vi "Set Build Specification Name.vi"(8 "error in (no error)":errorcluster, 10 "Build Specification Name":string, 11 "NI_AB_API_Build in":refnum<class "NI_AB_API_Build.lvclass">) -> (0 "error out":errorcluster, 3 "NI_AB_API_Build out":refnum<class "NI_AB_API_Build.lvclass">)   [LabVIEW 2020, in "NI_AB_API_Build.lvclass"]
uses:
  <vilib>/AppBuilder/AB_API/Build/NI_AB_API_Build.lvclass
  <vilib>/AppBuilder/AB_API/Build/NI_AB_API_Build.lvclass/NI_AB_API_Build.ctl
  <resource>/Framework/Providers/API/mxLvUpdateUI.ctl
  <vilib>/AppBuilder/AB_Classes/Build/AB_Build.lvclass
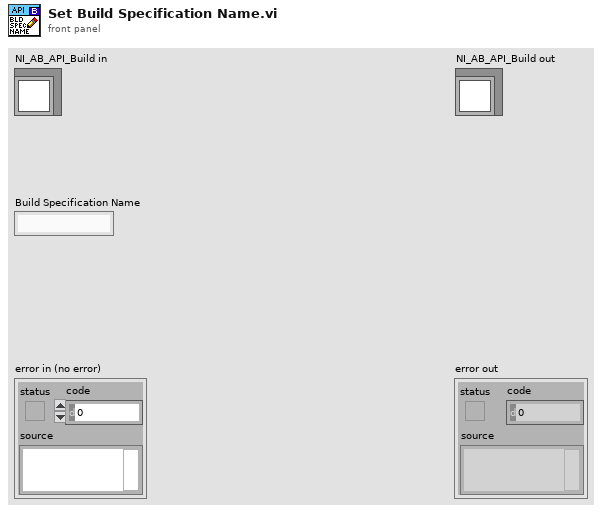
[diagram p1: front panel]
types:
  T1 = typedef "mxLvUpdateUI.ctl" = cluster{"Action":u32, "Optional param 1":string, "Optional param 2":i32, "Optional param 3":string}
  T2 = typedef "AB_Build.ctl" = cluster{"buildSpecName":string, "buildSpecDescription":string, "destinations":refnum<class "AB_Destination.lvclass">[], "exclusionOption":T3, "defaultLanguage":string, "supportedLanguages":string[], "excludedDirectories":path[], "buildContext":refnum<vi>, "buildObject":T4, "preview":bool, "programatic":bool, "progressBarEvents":T5, "userLog_Path":path, "preActionID":string, "preAction_Path":path, "postActionID":string, "postAction_Path":path, "eng_checkForBrokenVIs?":bool, "eng_verboseLinkerErrors?":bool, "localDest_Path":path, "targetDest_Path":path, "removeVIObject":u16, "cache":refnum<class "PreviewCache.lvclass">, "use cache":bool, "previewCache_ID":string, "buildCache_ID":string, "eng_TempLocalDest_Path":path, "eng_collectDependencies?":bool, "versionInfo":cluster{"buildVersion":cluster{"major":u16, "minor":u16, "patch":u16, "build":u16}, "autoIncrement":bool}, "eng_enableVIChecksums":bool}
  T3 = typedef "AB_Exclusion_Option.ctl" = cluster{"typedefs":bool, "polymorphicVIs":bool, "unusedLibraryItems":bool, "modifyLibraryFile":bool, "edit-timeDependencies":bool, "inlineVIs":bool, "dependent PPLs":bool, "dependent DLLs":bool}
  T4 = typedef "ItemRef.ctl" = u64
  T5 = typedef "provcom_ProgressBar_Events.ctl" = cluster{"newJob":refnum<user-event>, "newItem":refnum<user-event>, "errorMsg":T6, "cancel":refnum<user-event>}
  T6 = typedef "mxLvBuildError.ctl" = refnum<user-event>
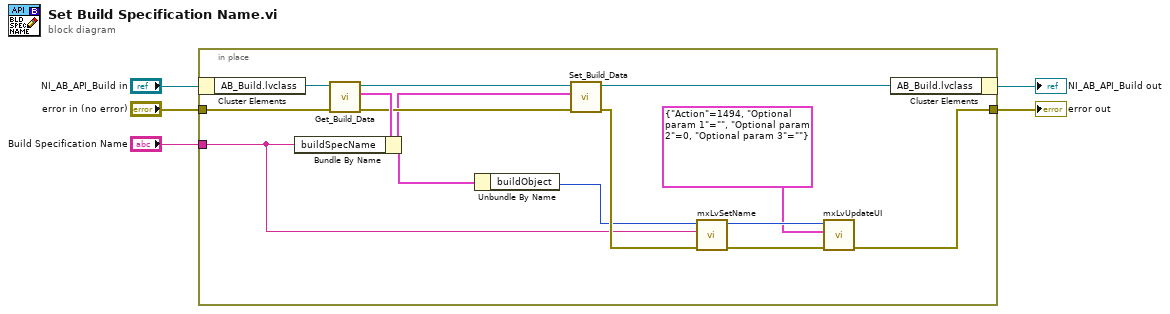
[diagram p0: block diagram]
diagram:
  n1 = in-place {
    in-place-border: [w11] -> w4
    in-place-border: "error in (no error)" -> [w19]
    in-place-border: "Build Specification Name" -> [w6]
    n2 = in-place-cluster #1("NI_AB_API_Build in") -> ("AB_Build.lvclass"=w14:refnum<class "AB_Build.lvclass">)
    n3 = call <vilib>:"Get_Build_Data.vi"("error in (no error)"=w19, "Class in"=w14) -> ("error out"=w16:errorcluster, "data"=w17:T2, "Class out"=w18:refnum<class "AB_Build.lvclass">)  [unwired: 7 out]
    n4 = Bundle By Name(cluster=w17, "buildSpecName"=w6) -> (w13:T2)
    n5 = Unbundle By Name(w13) -> ("buildObject"=w10:T4)
    n6 = call <vilib>:"Set_Build_Data.vi"("error in (no error)"=w16, "data"=w13, "Class in"=w18) -> ("error out"=w12:errorcluster, "Class out"=w15:refnum<class "AB_Build.lvclass">)  [unwired: 7 out]
    n7 = call <resource>:"mxLvSetName.vi"("error in"=w12, "Name"=w6, "Item"=w10) -> ("error out"=w8:errorcluster, "Item"=w9:T4)  [unwired: 7 in]
    n8 = call <resource>:"mxLvUpdateUI.vi"("error in"=w8, "Update UI Settings"=T1 {"Action"=1494, "Optional param 1"="", "Optional param 2"=0, "Optional param 3"=""}, "Item"=w9) -> ("error out"=w11:errorcluster)  [unwired: 7 in, 1 out]
    n9 = in-place-cluster #1("AB_Build.lvclass"=w15) -> (→"NI_AB_API_Build out":refnum<class "NI_AB_API_Build.lvclass">)
  }
  "error out" <- w4
